vi "Get All Tree Leaves.vi"(8 "error in":errorcluster, 11 "Tree in":refnum<class "Tree.lvclass">) -> (0 "error out":errorcluster, 1 "All Key Values":variant[](array[variant]), 2 "All Key Names":string[](array[string]), 3 "Tree out":refnum<class "Tree.lvclass">)   [LabVIEW 2019, in "Tree.lvclass"]
uses:
  Tree.lvclass
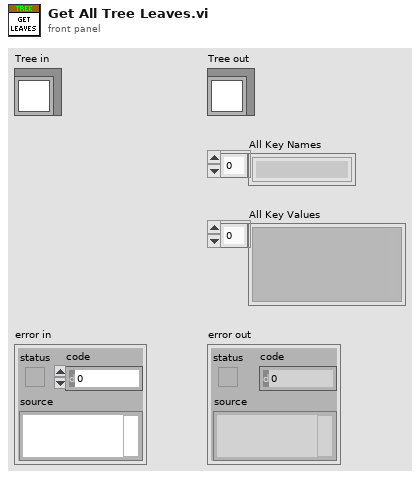
[diagram p1: front panel]
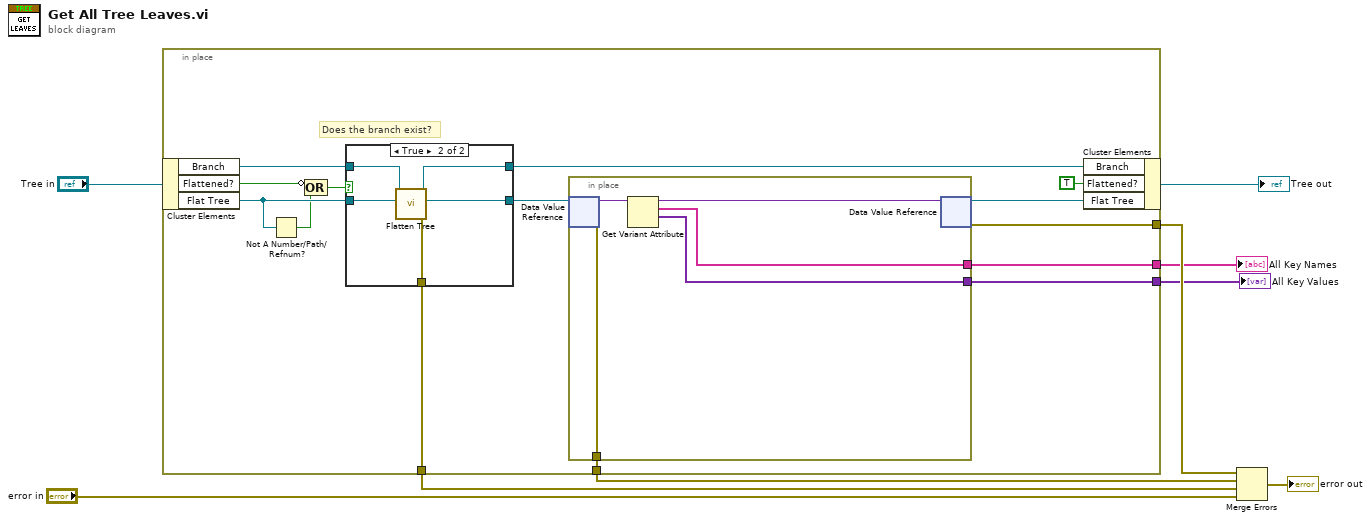
[diagram p0: block diagram]
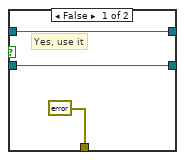
[diagram p2: hidden frame]
diagram:
  n1 = in-place {
    in-place-border: [w20] -> w5
    in-place-border: [w10] -> w3
    in-place-border: [w19] -> w4
    in-place-border: [w18] -> w2
    in-place-border: [w17] -> w1
    # "Does the branch exist?"
    n2 = in-place-cluster #1("Tree in") -> ("Branch"=w15:refnum<data-value>, "Flattened?"=w13:bool, "Flat Tree"=w23:refnum<data-value>)
    n3 = Not A Number/Path/Refnum?(number/path/refnum=w23) -> (NaN/Path/Refnum?=w12:bool)
    n4 = Compound Arithmetic op=OR(invert w13, w12) -> (w11:bool)
    n5 = case shown="True" w11 {
      tunnel: w23 -> [w31 w36]
      tunnel: [w31 w35] -> w22
      tunnel: [errorcluster {"status"=FALSE, "code"=0, "source"=""} ("error out") w32] -> w10
      tunnel: w15 -> [w29 w34]
      tunnel: [w29 w33] -> w14
      frame False {
        # "Yes, use it"
      }
      frame True {
        n6 = call "Flatten Tree.vi"("Flat Tree In"=w36, "Branch In"=w34) -> ("error out"=w32:errorcluster, "Flat Tree Out"=w35:refnum<data-value>, "Branch Out"=w33:refnum<data-value>)  [unwired: 7 in]
      }
    }
    n7 = in-place {
      in-place-border: [w28] -> w19
      in-place-border: [w25] -> w18
      in-place-border: [w24] -> w17
      n8 = in-place-dvr #2(w22) -> (w27:variant, w28:errorcluster)
      n9 = Get Variant Attribute(Variant=w27) -> (duplicate Variant=w26:variant, names=w25:string[], values=w24:variant[])  [unwired: 3 in, 1 out]
      n10 = in-place-dvr #2(w26) -> (w21:refnum<data-value>, w20:errorcluster)
    }
    n11 = in-place-cluster #1("Branch"=w14, "Flattened?"=TRUE, "Flat Tree"=w21) -> (→"Tree out":refnum<class "Tree.lvclass">)
  }
  "All Key Names" <- w2
  "All Key Values" <- w1
  n12 = Merge Errors(w5, w4, w3, "error in") -> (→"error out":errorcluster)
